vi "Simulate Noisy AI.vi"(4 "Simulate Waveguide [T]":bool=TRUE, 6 "Waveguide Cluster":T1={"Vsource Index"=0, "Vsg Index"=1, "V+"=0, "V-"=0}, 8 "error in (no error)":errorcluster, 11 "Instrument.Lockin.lvlib:Instrument.DAQ.lvclass":refnum<class "Instrument.DAQ.lvclass">) -> (0 "error out":errorcluster, 2 "Noisy Signal Graph":waveform(dbl)[](graph), 3 "Instrument.Lockin.lvlib:Instrument.DAQ.lvclass":refnum<class "Instrument.DAQ.lvclass">)   [LabVIEW 2019, in "Instrument.Lockin.lvlib" / "Instrument.DAQ.lvclass"]
uses:
  Instrument.DAQ.lvclass
  DAQmx/DAQmx.lvclass
  C:/Users/ansom/Documents/GitHub/Multichannel-Lockin/src/DAQ/DAQ.lvclass
  C:/Program Files (x86)/National Instruments/LabVIEW 2019/vi.lib/JKI/JKI SMO/SMO/SMO.lvclass
  Waveguide Model/Waveguide Model--Cluster.ctl
panel:
  out "Signal Graph":waveform(dbl)[](graph)
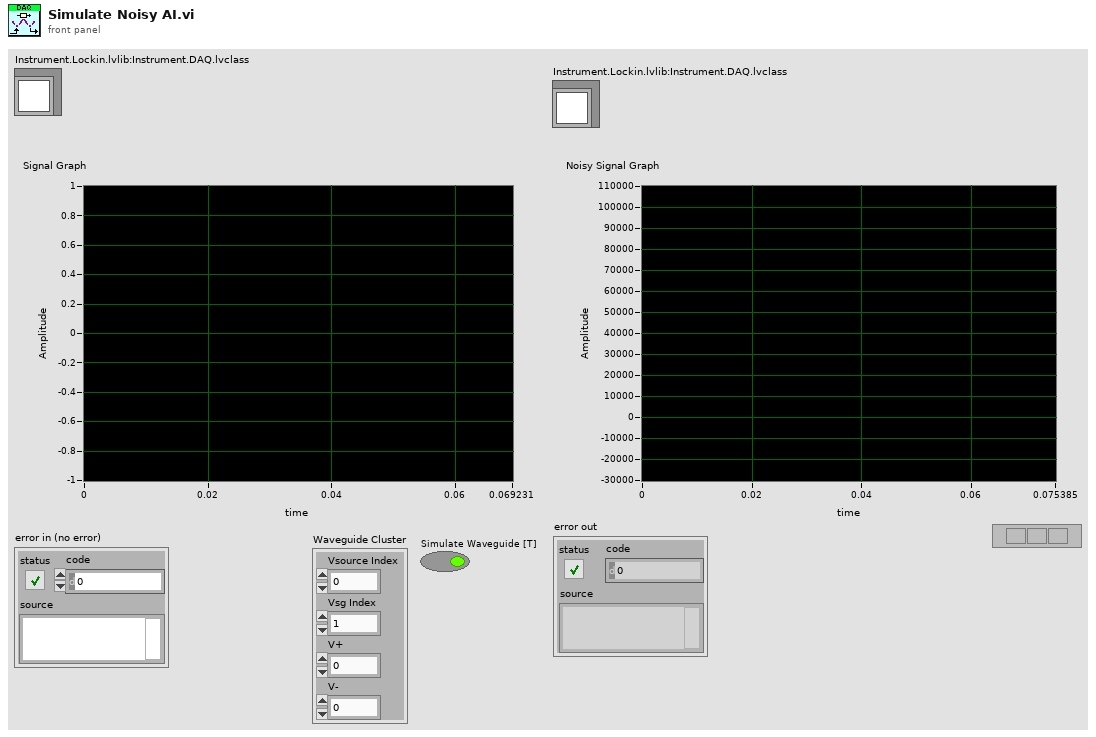
[diagram p1: front panel]
types:
  T1 = typedef "Instrument.Lockin.lvlib/Instrument.DAQ.lvclass/Waveguide Model--Cluster.ctl" = cluster{"Vsource Index":i32, "Vsg Index":i32, "V+":i32, "V-":i32}
  T2 = typedef "Instrument.Lockin.lvlib/Instrument.DAQ.lvclass/Simulation Mode--enum.ctl" = enum16{"AI = HW simulated", "AI = noise*AO", "AI = waveguide"}
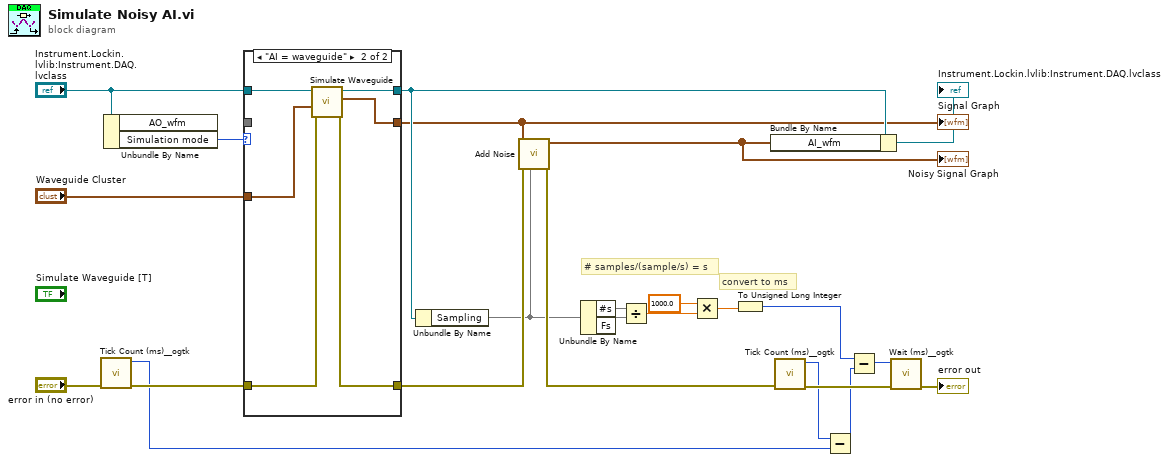
[diagram p0: block diagram]
diagram:
  # "convert to ms"
  # "# samples/(sample/s) = s"
  n1 = call <userlib>:"Tick Count (ms)__ogtk.vi"("error in (no error)"="error in (no error)") -> ("error out"=w11:errorcluster, "millisecond timer value"=w9:u32)  [unwired: 9 in]
  n2 = Unbundle By Name("Instrument.Lockin.lvlib:Instrument.DAQ.lvclass") -> ("Simulation mode"=w7:T2)  [unwired: 1 out]
  n3 = case shown="\"AI = waveguide\"" w7 {
    tunnel: w11 -> [w26 w30]
    tunnel: [w26 w29] -> w8
    tunnel: [w25 w33] -> w3
    tunnel: "Waveguide Cluster" -> [_ w28]
    tunnel: _ -> [w25 _]
    tunnel: "Instrument.Lockin.lvlib:Instrument.DAQ.lvclass" -> [w27 w32]
    tunnel: [w27 w31] -> w5
    frame "AI = noise*AO", Default {
    }
    frame "AI = waveguide" {
      n4 = call "Simulate Waveguide.vi"("error in (no error)"=w30, "Waveguide Cluster"=w28, "DAQmx in"=w32) -> ("error out"=w29:errorcluster, "AI []"=w33:waveform(dbl)[], "DAQmx out"=w31:refnum<class "DAQmx.lvclass">)  [unwired: 6 in]
    }
  }
  "Signal Graph" <- w3
  n5 = Unbundle By Name(w5) -> ("Sampling"=w2)
  n6 = call "Add Noise.vi"("Sampling"=w2, "error in (no error)"=w8, "AI []"=w3) -> ("error out"=w24:errorcluster, "AI + Noise"=w1:waveform(dbl)[])  [unwired: 7 in]
  "Noisy Signal Graph" <- w1
  n7 = Unbundle By Name(w2) -> ("#s"=w14, "Fs"=w15)
  n8 = Divide(x=w14, y=w15) -> (x/y=w18:dbl)
  n9 = Multiply(x=1000.0, y=w18) -> (x*y=w17:dbl)
  n10 = To Unsigned Long Integer(number=w17) -> (unsigned 32bit integer=w13:u32)
  n11 = Bundle By Name(cluster=w5, "AI_wfm"=w1) -> (→"Instrument.Lockin.lvlib:Instrument.DAQ.lvclass":refnum<class>)
  n12 = call <userlib>:"Tick Count (ms)__ogtk.vi"("error in (no error)"=w24) -> ("error out"=w23:errorcluster, "millisecond timer value"=w19:u32)  [unwired: 9 in]
  n13 = Subtract(x=w19, y=w9) -> (x-y=w20:u32)
  n14 = Subtract(x=w13, y=w20) -> (x-y=w21:u32)
  n15 = call <userlib>:"Wait (ms)__ogtk.vi"("error in (no error)"=w23, "milliseconds to wait"=w21) -> ("error out"=→"error out":errorcluster)  [unwired: 8 in, 1 out]
